vi "getInfo_action.vi"(0 "HGF_IMAQDevice":refnum<class "HGF_IMAQDevice.lvclass">, 5 "error in (no error)":errorcluster) -> (13 "imageType":T1 items=["Grayscale (U8)", "Grayscale (I16)", "Grayscale (SGL)", "Complex (CSG)", "RGB (U32)", "HSL (U32)", "RGB (U64)", "Grayscale (U16)"], 14 "dup HGF_IMAQDevice":refnum<class "HGF_IMAQDevice.lvclass">, 15 "cameraName":string, 16 "controlMode":T2, 17 "videoMode":i32, 19 "error out":errorcluster)   [LabVIEW 2014, in "HGF_IMAQ.lvlib" / "HGF_IMAQDevice.lvclass"]
doc: "Return the name of camera."
uses:
  HGF_IMAQDevice.lvclass
  Control Mode.ctl
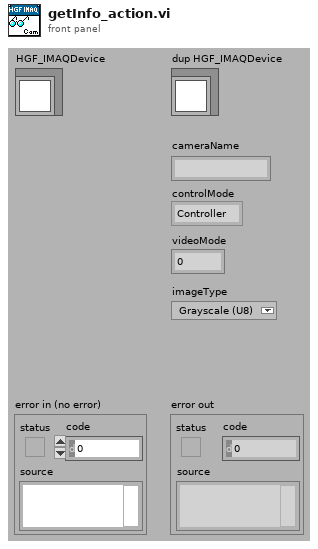
[diagram p1: front panel]
types:
  T1 = typedef "Image Type" = u32
  T2 = typedef "HGF_IMAQ.lvlib/HGF_IMAQDevice.lvclass/Control Mode.ctl" = enum16{"Controller", "Listener"}
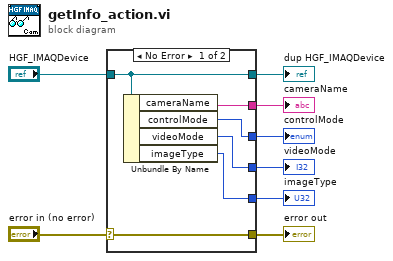
[diagram p0: block diagram]
diagram:
  n1 = case shown="No Error" "error in (no error)" {
    selector: "error in (no error)" -> [w14 w15]
    tunnel: [w14 w15] -> w7
    tunnel: [w13 w16] -> w5
    tunnel: "HGF_IMAQDevice" -> [w13 w16]
    tunnel: [w12 _] -> w4
    tunnel: [w11 _] -> w3
    tunnel: [w10 _] -> w2
    tunnel: [w9 _] -> w1
    frame No Error {
      n2 = Unbundle By Name(w13) -> ("cameraName"=w12:string, "controlMode"=w11:T2, "videoMode"=w10:i32, "imageType"=w9:T1)
    }
    frame Error {
    }
  }
  "error out" <- w7
  "dup HGF_IMAQDevice" <- w5
  "cameraName" <- w4
  "controlMode" <- w3
  "videoMode" <- w2
  "imageType" <- w1
